vi "File Name Message.vi"(8 "error in":errorcluster) -> (0 "error out":errorcluster, 2 "File Name Out":cluster{string, bool})   [LabVIEW 2016, in "CML UI.lvlib"]
doc: "<b>Note:</b> This VI was modified by the <b>Validate DQMH Module</b> tool to turn off automatic error handling."
uses:
  CML UI.lvlib
panel:
  in  "Cancel Button":bool
  in  "String input":string
  in  "OK Button":bool
  # "Enter File Name"
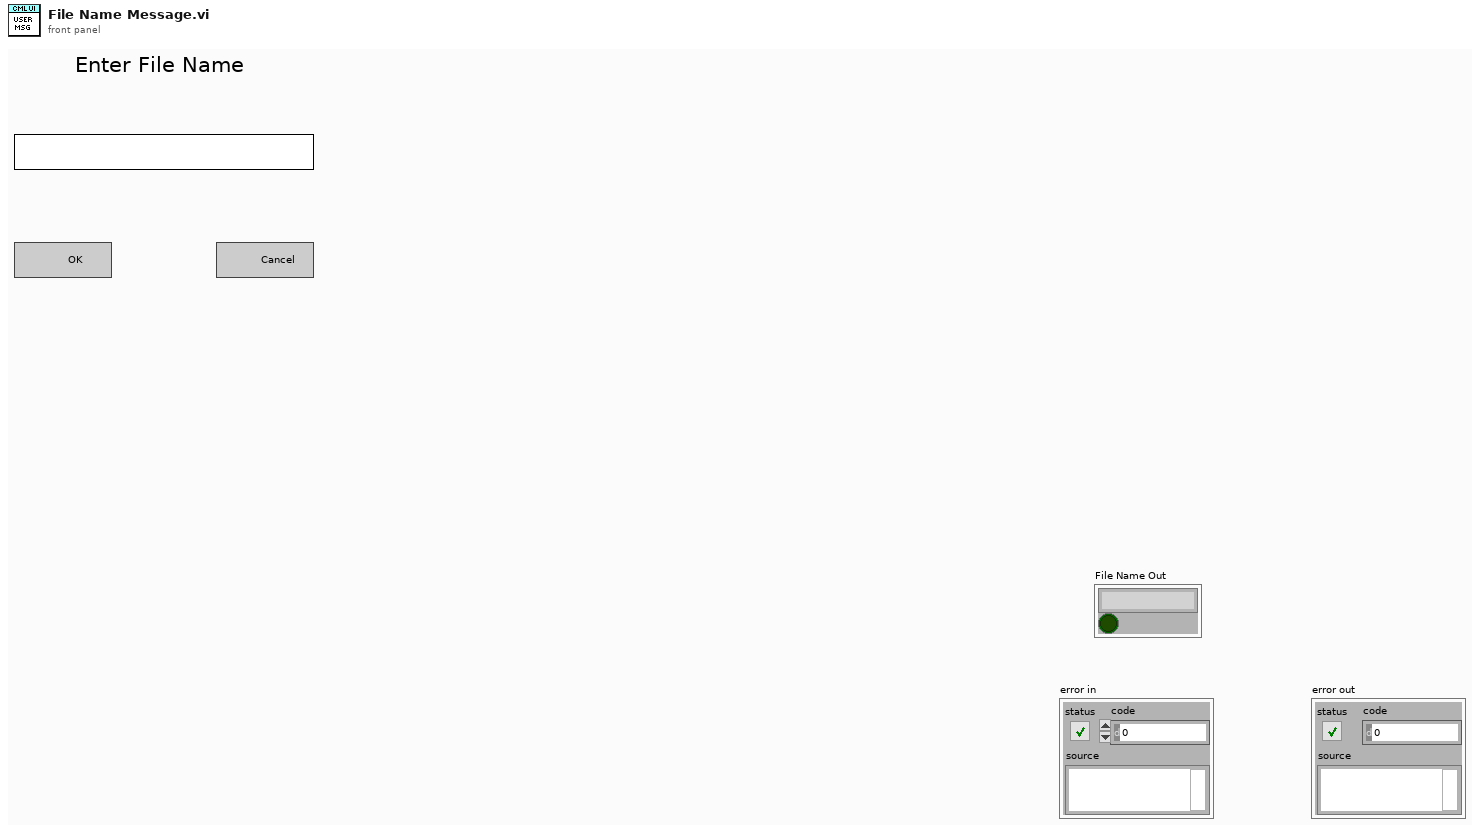
[diagram p1: front panel]
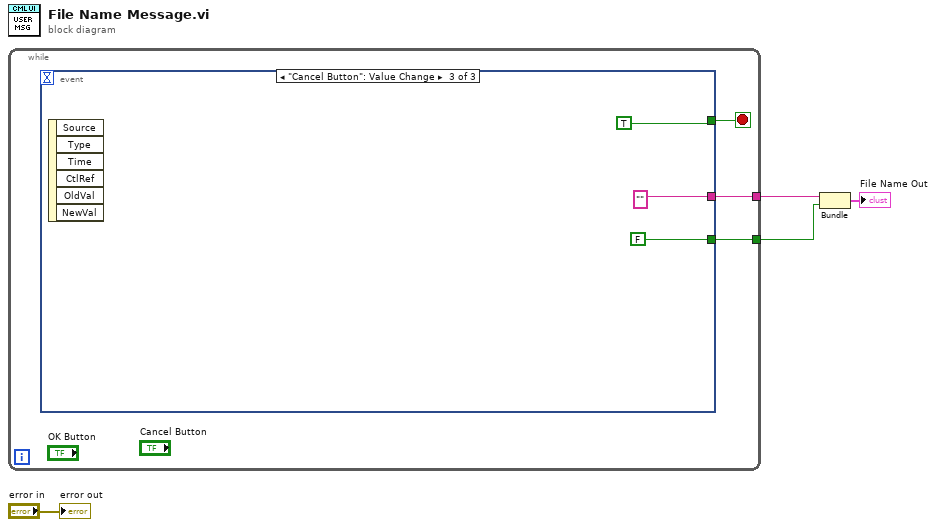
[diagram p0: block diagram]
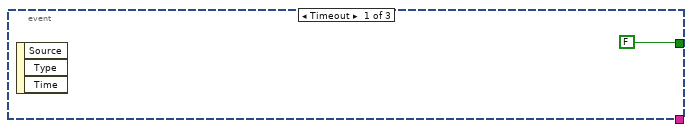
[diagram p2: hidden frame]
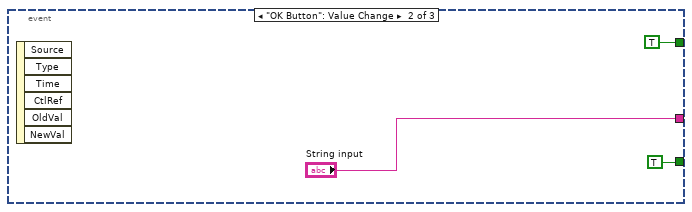
[diagram p3: hidden frame]
diagram:
  n1 = while {
    tunnel: [w6] -> w3
    tunnel: [w5] -> w2
    stop <- w7 stop-if-true
    n2 = event shown="[2] \"Cancel Button\": Value Change" {
      selector: _ -> [_ _ _]
      dyn-events: _ -> [_ _ _]
      timeout: _ -> [_ _ _]
      tunnel: [FALSE TRUE TRUE] -> w7
      tunnel: [_ "String input" ""] -> w6
      tunnel: [_ TRUE FALSE] -> w5
      event Timeout {
        n3 = event-data() -> ()  [unwired: 1 in, 3 out]
      }
      event "OK Button": Value Change {
        n4 = event-data() -> ()  [unwired: 1 in, 6 out]
      }
      event "Cancel Button": Value Change {
        n5 = event-data() -> ()  [unwired: 1 in, 6 out]
      }
    }
  }
  n6 = Bundle("String input"=w3, w2) -> (→"File Name Out":cluster{"String input":string, bool})  [unwired: 1 in]
  "error out" <- "error in"
